vi "Register Controller.vi"(5 "Control Panel Path":path, 6 "error in (no error)":errorcluster, 8 "Controller Type":T1, 9 "Controller Array in":refnum<class "Controller Array.lvclass">) -> (0 "error out":errorcluster, 1 "New Controller out":refnum<class "Generic Plugin.lvclass">, 2 "Registered?":bool, 3 "Controller Array out":refnum<class "Controller Array.lvclass">)   [LabVIEW 2020, in "RxnRover.lvlib" / "Controller Array.lvclass"]
doc: "Given a control type and name, load a controller of that name and add it to the end of the controller array."
uses:
  Controller Array.lvclass
  Controller/Controller Type.ctl
  Controller/Generic Plugin.lvclass
  <userlib>/RxnRover/DynamicReentrant/src/Type Defs/Message.ctl
  <userlib>/RxnRover/DynamicReentrant/Dynamic Reentrant.lvlib
panel:
  in  "Receiving Queue":refnum<queue>
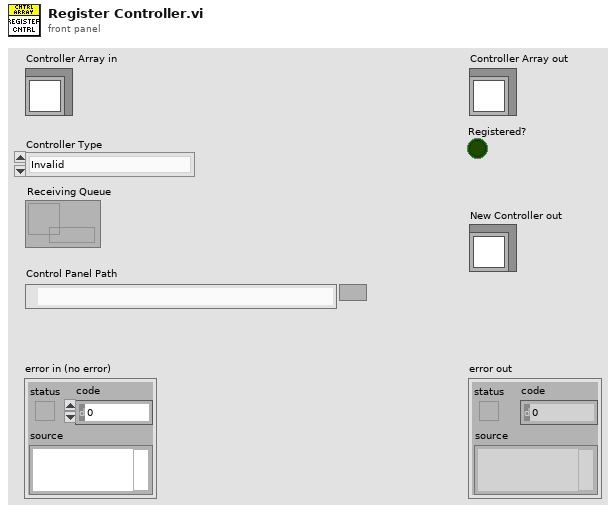
[diagram p1: front panel]
types:
  T1 = typedef "RxnRover.lvlib/Generic Plugin.lvclass/Controller Type.ctl" = enum16{"Invalid", "Temperature Controller", "Pump Controller", "Syringe Pump", "Generic Optimizer", "LC Parser"}
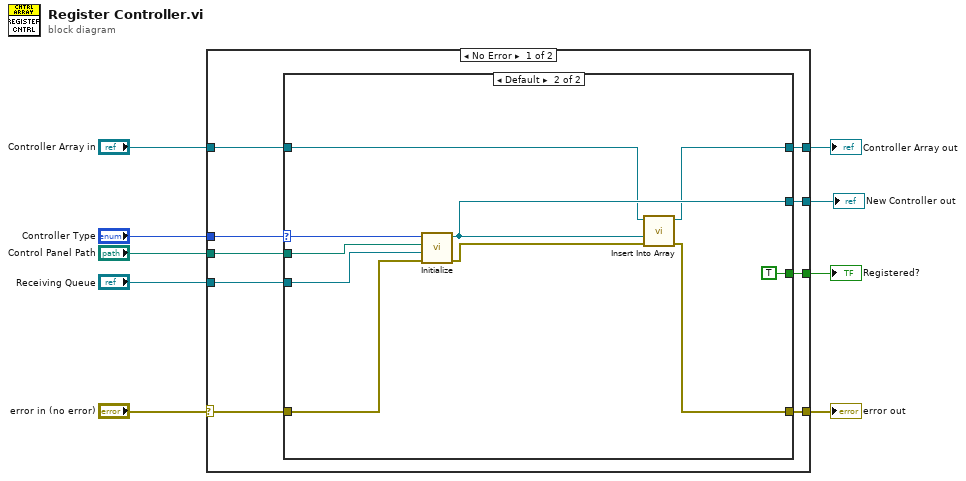
[diagram p0: block diagram]
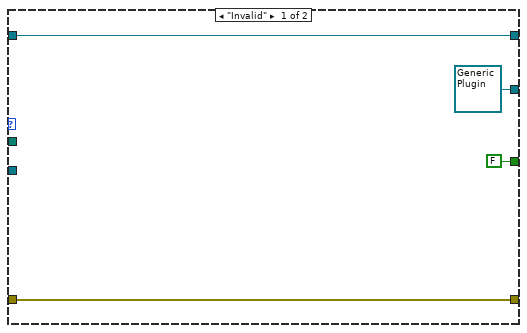
[diagram p2: hidden frame]
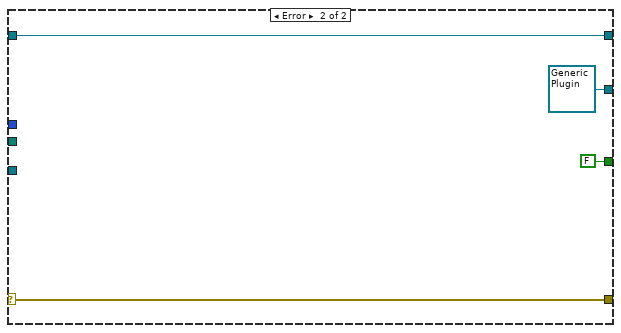
[diagram p3: hidden frame]
diagram:
  n1 = case shown="No Error" "error in (no error)" {
    selector: "error in (no error)" -> [w14 w36]
    tunnel: [w16 w36] -> w8
    tunnel: [w18 w35] -> w6
    tunnel: "Controller Array in" -> [w17 w35]
    tunnel: "Controller Type" -> [w12 _]
    tunnel: [w15 FALSE] -> w4
    tunnel: [w13 refnum<class "Generic Plugin.lvclass"> refnum ("controller out")] -> w3
    tunnel: "Control Panel Path" -> [w11 _]
    tunnel: "Receiving Queue" -> [w10 _]
    frame No Error {
      n2 = case shown="Default" w12 {
        selector: w12 -> [_ w28]
        tunnel: [w22 w24] -> w18
        tunnel: w17 -> [w22 w25]
        tunnel: [w19 w32] -> w16
        tunnel: [FALSE TRUE] -> w15
        tunnel: w14 -> [w19 w30]
        tunnel: [refnum<class "Generic Plugin.lvclass"> refnum ("controller out") w31] -> w13
        tunnel: w11 -> [_ w26]
        tunnel: w10 -> [_ w23]
        frame "Invalid" {
        }
        frame Default {
          n3 = call "Initialize.vi"("error in (no error)"=w30, "Receiving Queue"=w23, "Control Panel Path"=w26, "Controller Type"=w28) -> ("error out"=w29:errorcluster, "Plugin Server out"=w31:refnum<class "Generic Plugin.lvclass">)  [unwired: 5 in, 1 out]
          n4 = call "Insert Into Array.vi"("error in (no error)"=w29, "new element"=w31, "Controller Array in"=w25) -> ("error out"=w32:errorcluster, "Controller Array out"=w24:refnum<class "Controller Array.lvclass">)  [unwired: 2 in, 1 out]
        }
      }
    }
    frame Error {
    }
  }
  "error out" <- w8
  "Controller Array out" <- w6
  "Registered?" <- w4
  "New Controller out" <- w3
